vi "Memory.Pointer.Parameter Check.Offset.vi"(7 "calling vi name":string, 8 "error in (no error)":errorcluster, 10 "offset":u64 format="%d bytes", 11 "Pointer in":refnum<class "Memory.Pointer.Void.lvclass">) -> (0 "error out":errorcluster, 2 "offset out":u64 format="%d bytes", 3 "Pointer out":refnum<class "Memory.Pointer.Void.lvclass">)   [LabVIEW 2016, in "Memory.Pointer.Void.lvclass"]
uses:
  Memory.Pointer.Void.lvclass
  Pointer/Typedefs/Memory.Pointer.Parameters.ctl
  Pointer/Memory.Pointer.lvclass
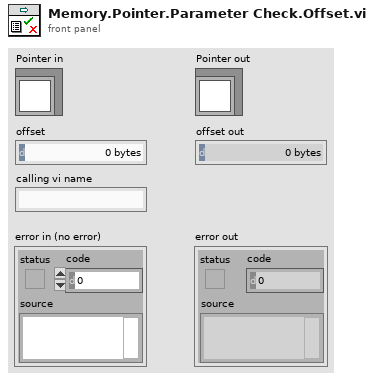
[diagram p1: front panel]
types:
  T1 = typedef "Memory Manager.lvlib/Memory.Pointer.lvclass/Memory.Pointer.Parameters.ctl" = enum16{"offset", "length", "size", "subset"}
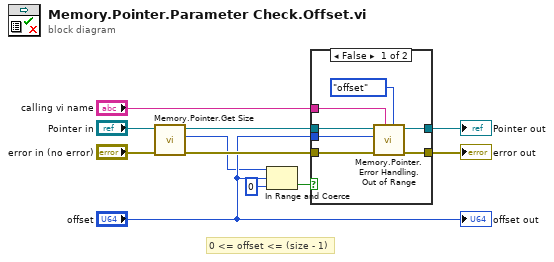
[diagram p0: block diagram]
diagram:
  # "0 <= offset <= (size - 1)"
  n1 = call "Memory.Pointer.Get Size.vi"("error in (no error)"="error in (no error)", "Pointer in"="Pointer in") -> ("error out"=w8:errorcluster, "size"=w1:u64, "Pointer out"=w11:refnum<class "Memory.Pointer.Void.lvclass">)  [unwired: 7 in]
  n2 = In Range and Coerce(upper limit=w1, x="offset", lower limit=u64 0) -> (In Range?=w10:bool)  [unwired: 1 out]
  n3 = case shown="False" w10 {
    tunnel: [w18 w20] -> w4
    tunnel: "calling vi name" -> [w17 _]
    tunnel: w8 -> [w16 w20]
    tunnel: "offset" -> [w14 _]
    tunnel: w11 -> [w13 w19]
    tunnel: [w12 w19] -> w3
    frame False {
      n4 = call "Memory.Pointer.Error Handling.Out of Range.vi"("parameter"=Memory.Pointer.Parameters."offset", "source vi name"=w17, "error in (no error)"=w16, "value"=w14, "pointer in"=w13) -> ("error out"=w18:errorcluster, "pointer out"=w12:refnum<class "Memory.Pointer.lvclass">)  [unwired: 5 in]
    }
    frame True {
    }
  }
  "error out" <- w4
  "Pointer out" <- w3
  "offset out" <- "offset"
